vi "Settings.vi"(8 "error in (no error)":errorcluster, 10 "shutdown":refnum<user-event>, 11 "Modules":T1) -> (0 "error out":errorcluster)   [LabVIEW 2025]
uses:
  <vilib>/Handler Framework/CmdQueue/Enqueue Single.vi
  <vilib>/Handler Framework/Handler Framework.lvlib
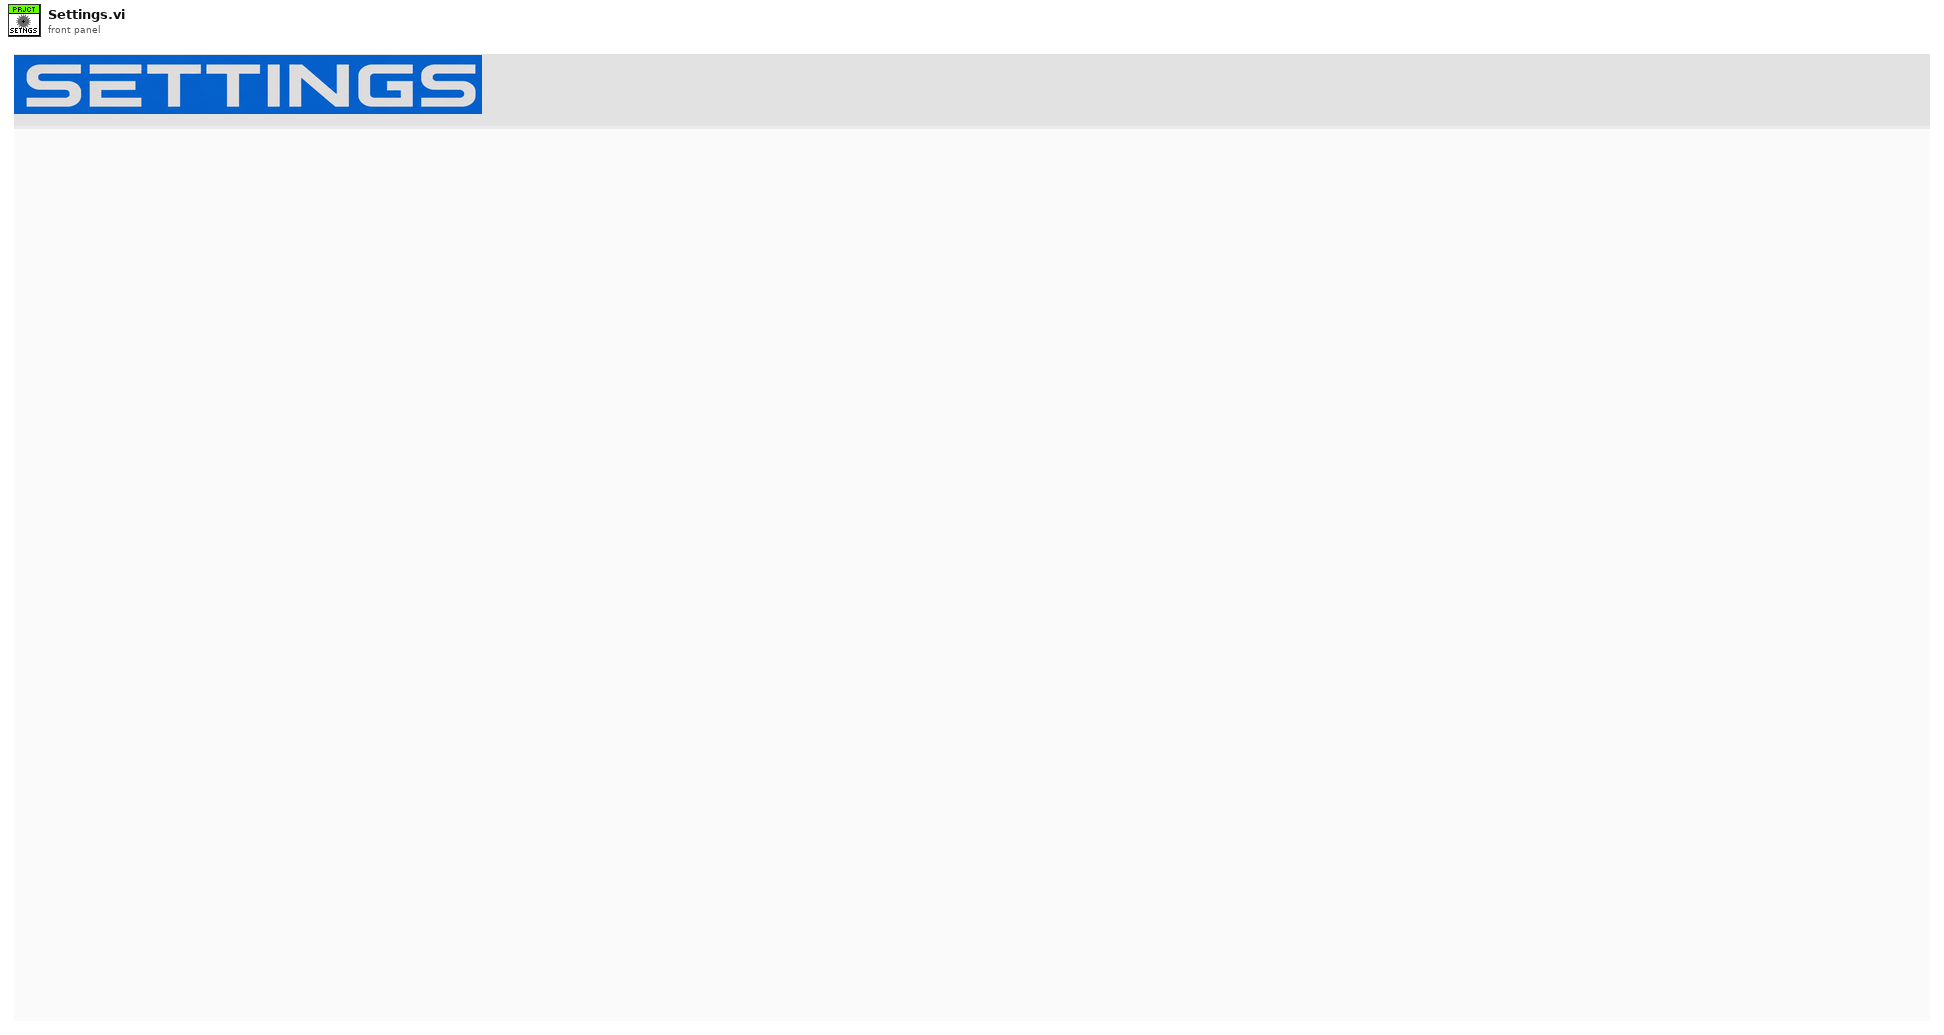
[diagram p1: front panel]
types:
  T1 = cluster{"Module IDs":i32[], "Module Names":string[]}
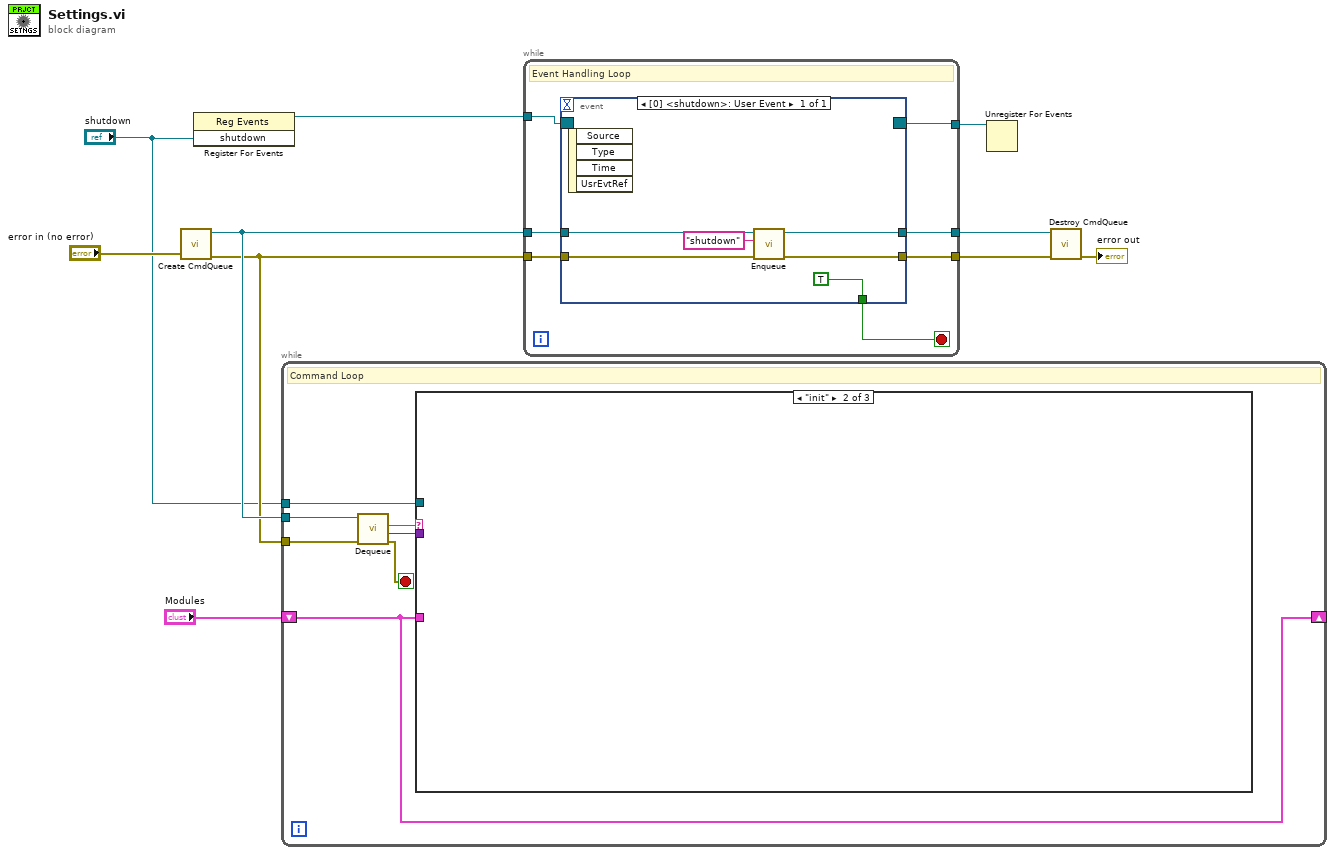
[diagram p0: block diagram]
diagram:
  n1 = call <vilib>:"Create CmdQueue.vi"("error in (no error)"="error in (no error)") -> ("error out"=w7:errorcluster, "CmdQueue out"=w8:refnum<queue>)  [unwired: 9 in]
  n2 = register-events("shutdown") -> (reference out=w6:refnum<event-registration>)  [unwired: 2 in, 1 out]
  n3 = while {
    tunnel: w8 -> [w17]
    tunnel: w7 -> [w13]
    tunnel: "shutdown" -> [w12]
    shift-right: [w11] -> _
    shift-left: "Modules" -> [w11]
    stop <- w14 stop-if-true
    # "Command Loop"
    n4 = call <vilib>:"Dequeue.vi"("error in (no error)"=w13, "CmdQueue in"=w17) -> ("error out"=w14:errorcluster, "value"=w15:variant, "cmd"=w16:string)  [unwired: 5 in, 2 out]
    n5 = case shown="\"init\"" w16 {
      tunnel: w15 -> [_ _ _]
      tunnel: w12 -> [_ _ _]
      tunnel: w11 -> [_ _ _]
      frame "False", Default {
      }
      frame "init" {
      }
      frame "shutdown" {
      }
    }
  }
  n6 = while {
    tunnel: w8 -> [w24]
    tunnel: [w23] -> w10
    tunnel: w7 -> [w22]
    tunnel: [w21] -> w9
    tunnel: w6 -> [w19]
    tunnel: [w18] -> w5
    stop <- w20 stop-if-true
    # "Event Handling Loop"
    n7 = event shown="[0] <shutdown>: User Event" {
      selector: w19 -> [_]
      dyn-events: [_] -> w18
      timeout: _ -> [_]
      tunnel: w24 -> [w30]
      tunnel: [w29] -> w23
      tunnel: w22 -> [w28]
      tunnel: [w27] -> w21
      tunnel: [TRUE ("Discard?")] -> w20
      event User Event {
        n8 = event-data() -> ()  [unwired: 1 in, 4 out]
        n9 = call-poly <vilib>:"Enqueue.vi"("error in (no error)"=w28, "Command"="shutdown", "CmdQueue in"=w30) -> ("error out"=w27:errorcluster, "CmdQueue out"=w29:refnum<queue>)  [unwired: 7 in]
      }
    }
  }
  n10 = Unregister For Events(event registration refnum=w5) -> ()  [unwired: 1 in, 1 out]
  n11 = call <vilib>:"Destroy CmdQueue.vi"("error in (no error)"=w9, "CmdQueue in"=w10) -> ("error out"=→"error out":errorcluster)  [unwired: 9 in]
